vi "Global.vi"() -> ()   [LabVIEW 2010, in "TDMS to ASCII Convert.lvlib"]
uses:
  TDMS to ASCII Convert.lvlib
panel:
  out "Settings":refnum<vi>[](array[refnum])
  out "Abort Flag":bool
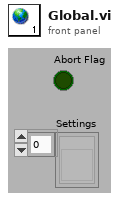
[diagram p1: front panel]
diagram:
